vi "intepret.vi"(8 "error in (no error)":errorcluster, 10 "context":string, 11 "TerminalExpression in":refnum<class "TerminalExpression.lvclass">) -> (0 "error out":errorcluster, 2 "result":bool, 3 "TerminalExpression out":refnum<class "TerminalExpression.lvclass">)   [LabVIEW 2017, in "TerminalExpression.lvclass"]
uses:
  TerminalExpression.lvclass
  TerminalExpression.lvclass/TerminalExpression.ctl
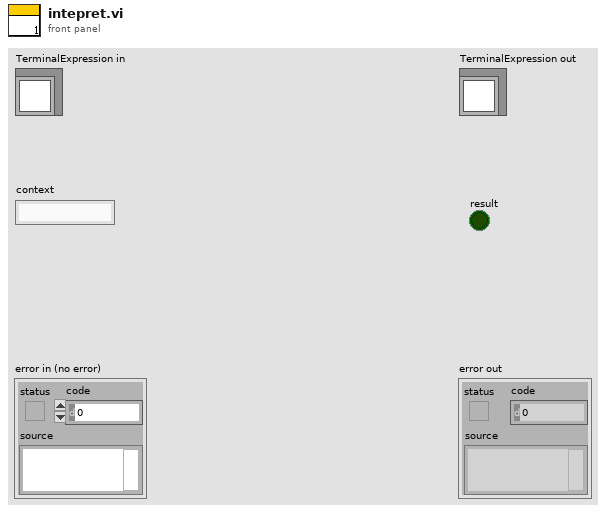
[diagram p1: front panel]
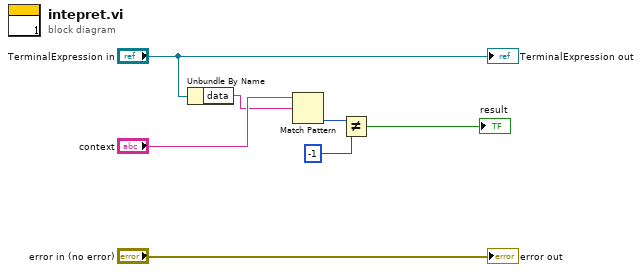
[diagram p0: block diagram]
diagram:
  n1 = Unbundle By Name("TerminalExpression in") -> ("data"=w1:string)
  n2 = Match Pattern(string="context", regular expression=w1) -> (offset past match=w5:i32)  [unwired: 1 in, 3 out]
  n3 = Not Equal?(x=w5, y=-1) -> (x != y?=→"result":bool)
  "error out" <- "error in (no error)"
  "TerminalExpression out" <- "TerminalExpression in"
